vi "Untitled 2.vi"() -> ()   [LabVIEW 2017]
panel:
  out "TempLabels":string[][](array[string])
  out "FuelLabels":T1(array[cluster])
  out "FuelData":bool=TRUE
  out "TempData":bool=TRUE
  out "Temperatures":dbl[][](array[numeric])
  out "FuelFlows":dbl[][](array[numeric])
  in  "f_q":dbl[][](array[numeric])
  in  "temp typedef":dbl[][](array[numeric])
  in  "f_q 2":dbl[][](array[numeric])
  in  "Array 5":dbl[][](array[numeric])
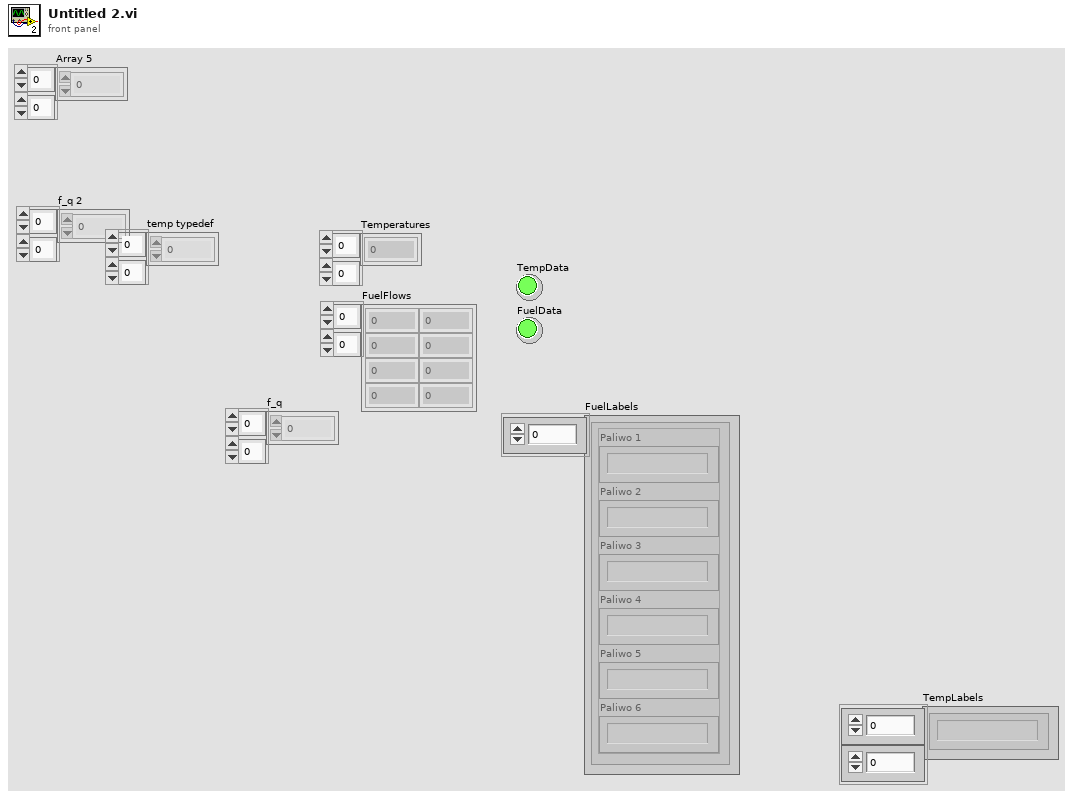
[diagram p1: front panel]
types:
  T1 = cluster{"Paliwo 1":string, "Paliwo 2":string, "Paliwo 3":string, "Paliwo 4":string, "Paliwo 5":string, "Paliwo 6":string}[]
  T2 = cluster{"Termometr 1":string, "Termometr 2":string, "Termometr 3":string, "Termometr 4":string, "Termometr 5":string, "Termometr 6":string, "Termometr 7":string, "Termometr 8":string, "Termometr 9":string, "Termometr 10":string}
  T3 = cluster{"Paliwo 1":string, "Paliwo 2":string, "Paliwo 3":string, "Paliwo 4":string, "Paliwo 5":string, "Paliwo 6":string}
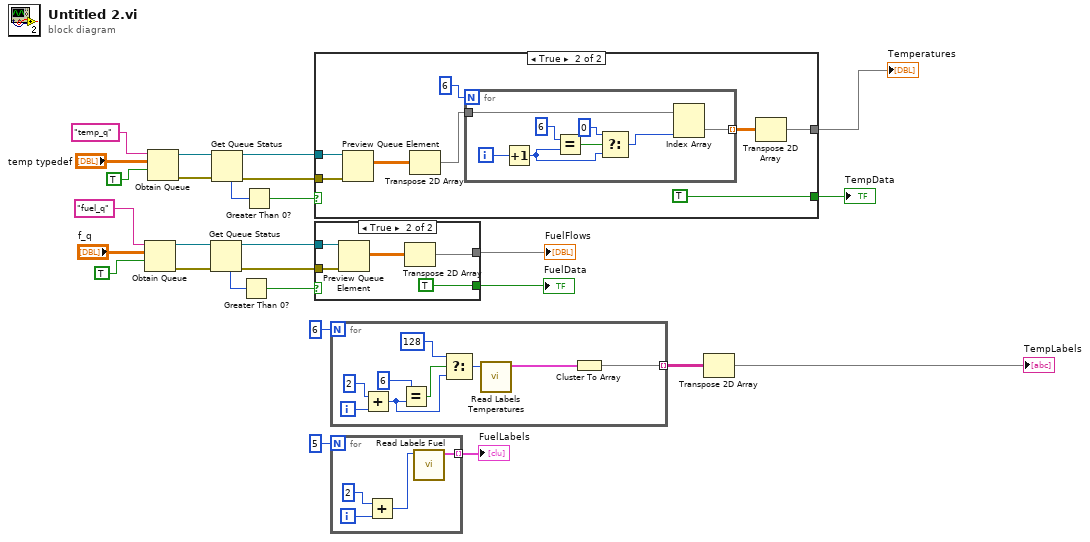
[diagram p0: block diagram]
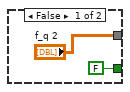
[diagram p2: hidden frame]
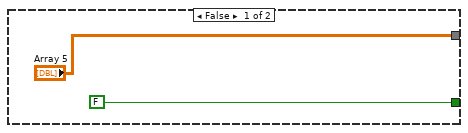
[diagram p3: hidden frame]
diagram:
  n1 = Obtain Queue(name (unnamed)="fuel_q", element data type="f_q", create if not found? (T)=TRUE) -> (queue out=w13:refnum<queue>, error out=w12:errorcluster)  [unwired: 2 in, 1 out]
  n2 = Obtain Queue(name (unnamed)="temp_q", element data type="temp typedef", create if not found? (T)=TRUE) -> (queue out=w10:refnum<queue>, error out=w11:errorcluster)  [unwired: 2 in, 1 out]
  n3 = Get Queue Status(queue=w13, error in (no error)=w12) -> (queue out=w20:refnum<queue>, error out=w21:errorcluster, # elements in queue=w23:i32)  [unwired: 1 in, 5 out]
  n4 = Get Queue Status(queue=w10, error in (no error)=w11) -> (queue out=w25:refnum<queue>, error out=w26:errorcluster, # elements in queue=w27:i32)  [unwired: 1 in, 5 out]
  n5 = Greater Than 0?(x=w23) -> (x > 0?=w22:bool)
  n6 = Greater Than 0?(x=w27) -> (x > 0?=w24:bool)
  n7 = case shown="True" w24 {
    tunnel: w26 -> [_ w36]
    tunnel: w25 -> [_ w37]
    tunnel: ["Array 5" w30] -> w2
    tunnel: [FALSE TRUE] -> w7
    frame False {
    }
    frame True {
      n8 = Preview Queue Element(queue=w37, error in (no error)=w36) -> (element=w34:dbl[][])  [unwired: 1 in, 3 out]
      n9 = Transpose 2D Array(2D array=w34) -> (transposed array=w32:dbl[][])
      n10 = for {
        N: 6 -> [_]
        tunnel: w32 -> [w44]
        tunnel: [w43] -> w31 mode=indexing
        i -> [w45]
        n11 = Increment(x=w45) -> (x+1=w38:i32)
        n12 = Equal?(x=6 ("y"), y=w38) -> (x = y?=w42:bool)
        n13 = Select(t=0, s=w42, f=w38) -> (s? t:f=w39:i32)
        n14 = Index Array(array=w44, index (col)=w39) -> (element=w43:dbl[])  [unwired: 1 in]
      }
      n15 = Transpose 2D Array(2D array=w31) -> (transposed array=w30:dbl[][])
    }
  }
  "Temperatures" <- w2
  "TempData" <- w7
  n16 = case shown="True" w22 {
    tunnel: w20 -> [_ w52]
    tunnel: w21 -> [_ w51]
    tunnel: ["f_q 2" w48] -> w9
    tunnel: [FALSE TRUE] -> w8
    frame False {
    }
    frame True {
      n17 = Preview Queue Element(queue=w52, error in (no error)=w51) -> (element=w49:dbl[][])  [unwired: 1 in, 3 out]
      n18 = Transpose 2D Array(2D array=w49) -> (transposed array=w48:dbl[][])
    }
  }
  "FuelFlows" <- w9
  "FuelData" <- w8
  n19 = for {
    N: 6 -> [_]
    tunnel: [w53] -> w3 mode=indexing
    i -> [w61]
    n20 = Add(x=2, y=w61) -> (x+y=w56:i32)
    n21 = Equal?(x=6, y=w56) -> (x = y?=w57:bool)
    n22 = Select(t=128, s=w57, f=w56) -> (s? t:f=w59:i32)
    n23 = call "Read Labels Temperatures.vi"("Slave ID"=w59) -> ("Etykiety T1-10"=w54:T2)  [unwired: 10 in]
    n24 = Cluster To Array(cluster=w54) -> (array=w53:string[])
  }
  n25 = for {
    N: 5 -> [_]
    tunnel: [w62] -> w5 mode=indexing
    i -> [w65]
    n26 = Add(x=2, y=w65) -> (x+y=w63:i32)
    n27 = call "Read Labels Fuel.vi"("Slave ID"=w63) -> ("Etykiety P1-6"=w62:T3)  [unwired: 10 in]
  }
  "FuelLabels" <- w5
  n28 = Transpose 2D Array(2D array=w3) -> (transposed array=→"TempLabels":string[][])
